vi "Find File By Name.vi"(6 "Path (If Folder Path is empty)":enum16{"vi.lib", "user.lib", "instr.lib"}(ring)=enum."instr.lib", 8 "error in (no error)":errorcluster, 10 "File Name":string, 11 "Folder Path":path) -> (0 "error out":errorcluster, 3 "File Path":path)   [LabVIEW 2016]
uses:
  <vilib>/Utility/error.llb/Error Cluster From Error Code.vi
  <vilib>/ErrorRing/Error Ring.xnode
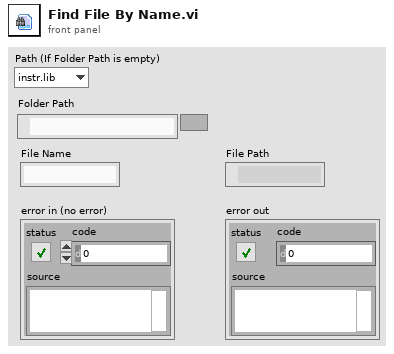
[diagram p1: front panel]
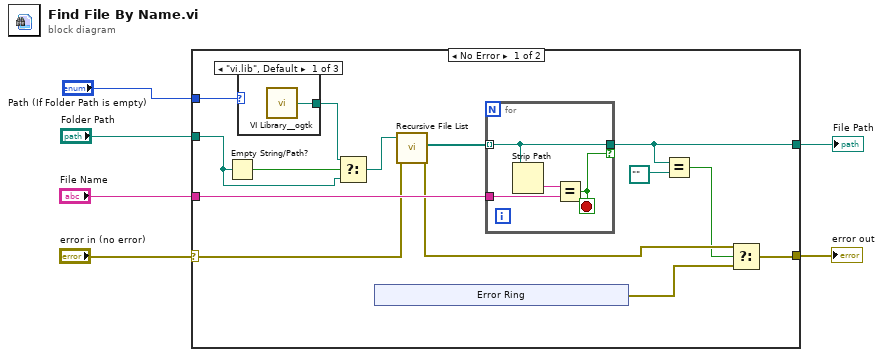
[diagram p0: block diagram]
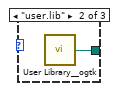
[diagram p2: hidden frame]
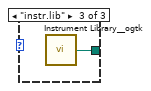
[diagram p3: hidden frame]
diagram:
  n1 = case shown="No Error" "error in (no error)" {
    selector: "error in (no error)" -> [w18 w32]
    tunnel: [w13 w32] -> w6
    tunnel: [w16 _] -> w5
    tunnel: "File Name" -> [w20 _]
    tunnel: "Folder Path" -> [w9 _]
    tunnel: "Path (If Folder Path is empty)" -> [w7 _]
    frame No Error {
      n2 = Empty String/Path?(string/path=w9) -> (empty?=w11:bool)
      n3 = case shown="\"vi.lib\", Default" w7 {
        tunnel: [w21 w22 w23] -> w10
        frame "vi.lib", Default {
          n4 = call <userlib>:"VI Library__ogtk.vi"() -> ("VI Library (+ Relative)"=w21:path)  [unwired: 1 in]
        }
        frame "user.lib" {
          n5 = call <userlib>:"User Library__ogtk.vi"() -> ("User Library (+ Relative)"=w22:path)  [unwired: 1 in]
        }
        frame "instr.lib" {
          n6 = call <userlib>:"Instrument Library__ogtk.vi"() -> ("Instrument Library (+ Relative)"=w23:path)  [unwired: 1 in]
        }
      }
      n7 = Select(t=w10, s=w11, f=w9) -> (s? t:f=w8:path)
      n8 = xnode "Error Ring"() -> ("error out"=w14:errorcluster)
      n9 = call <vilib>:"Recursive File List.vi"("error in (no error)"=w18, "Folder Path"=w8) -> ("error out"=w15:errorcluster, "All Files in Dir"=w19:path[])  [unwired: 5 in, 3 out]
      n10 = for {
        tunnel: w19 -> [w29] mode=indexing
        tunnel: w20 -> [w30]
        tunnel: [w29] -> w16 if=w28
        stop <- w28 stop-if-true
        n11 = Strip Path(path=w29) -> (name=w31:string)  [unwired: 1 out]
        n12 = Equal?(x=w31, y=w30) -> (x = y?=w28:bool)
      }
      n13 = Equal?(x=w16, y=path "") -> (x = y?=w12:bool)
      n14 = Select(t=w15, s=w12, f=w14) -> (s? t:f=w13:errorcluster)
    }
    frame Error {
    }
  }
  "error out" <- w6
  "File Path" <- w5
